vi "configure.vi"(8 "error in (no error)":errorcluster, 11 "user":string) -> (0 "error out":errorcluster, 2 "cancelled?":bool)   [LabVIEW 2010]
uses:
  components/Stage/GenericStage/GenericStage/GenericStage.lvclass
  components/ExperimentController/GenericExperimentController/GenericExperimentController/GenericExperimentController.lvclass
  components/ImagingMode/GenericImagingMode/GenericImagingMode/GenericImagingMode.lvclass
  components/Objective/GenericObjective/GenericObjective/GenericObjective.lvclass
  common/classes/ErrorController/ErrorController/class_data.vi
  common/classes/GenericComponent/GenericComponent/GenericComponent.lvclass
  common/classes/ErrorController/ErrorController/ErrorController.lvclass
panel:
  in  "Tab Control":T1(tab)
  in  "configure experiment controllers":bool
  in  "configure scan modes":bool
  in  "manageObjectivesButton":bool
  in  "configure objectives":bool
  in  "configure stage":bool
  in  "stage configuration":string(combo) caption="configuration"
  in  "stage path":path=path "C:/helioscan/plugins/scan_head/DL090202ScanHead/DL090202ScanHead/DL090202ScanHead.lvclass" caption="Component class path (.lvclass file)"
  in  "cancelButton":bool
  in  "save":bool
  # "HelioScan Main Configuration"
  # "ExperimentController components control the execution of individual scans. Here you can add ExperimentControllers, such that they can be selected from a drop-down menu in the main application. \n\nImportant: Note that some of the ExperimentControllers might require to be configured before you add them here."
  # "Each ImagingMode component controls a specific kind of image acquisition (e.g., video camera, intrinsic imaging, different laser-scanning-based ImagingModes, etc.). Here you can add ImagingModes, such that they can be selected from a drop-down menu in the main application. \n\nImportant: Note that you have to configure an ImagingMode before you can add it here."
  # "Objective components hold information about a specific microscope objective (e.g., magnification, manufacturer, etc.).\n\nImportant: Note that you have to configure an Objective component before you can add it here."
  # "The Stage component is responsible for controlling a motorised microscopy stage.\n\nNote: If you do not want to control a stage with HelioScan, just leave the input boxes below empty."
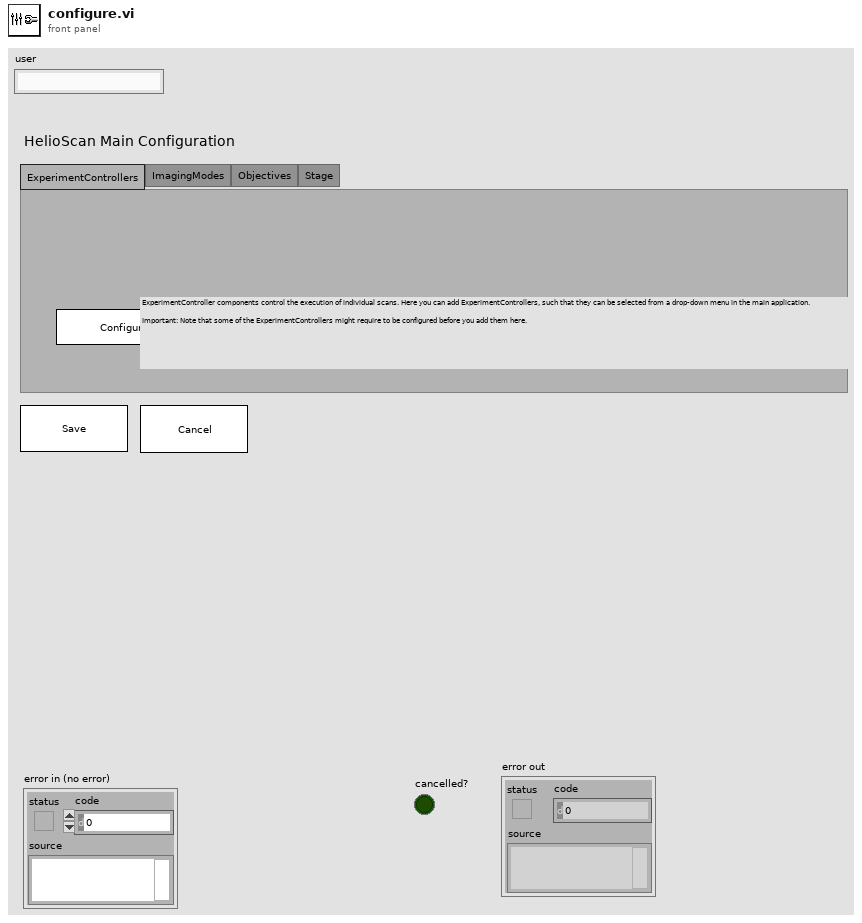
[diagram p1: front panel]
types:
  T1 = enum32{"ExperimentControllers", "ImagingModes", "Objectives", "Stage"}
  T2 = typedef "configuration_paths_cluster.ctl" = cluster{"base folder":path, "base folder for user":path, "component folder":path, "component file path":path, "main folder":path, "main file":path}
  T3 = typedef "top_level_config_cluster.ctl" = cluster{"experimentControllers":T4[], "default experimentController":string, "imagingModes":T4[], "default imagingMode":string, "stage":T4, "objectives":T4[], "default objective":string}
  T4 = typedef "plugin_specification.ctl" = cluster{"class path":string, "configuration":string, "label":string, "settings name":string}
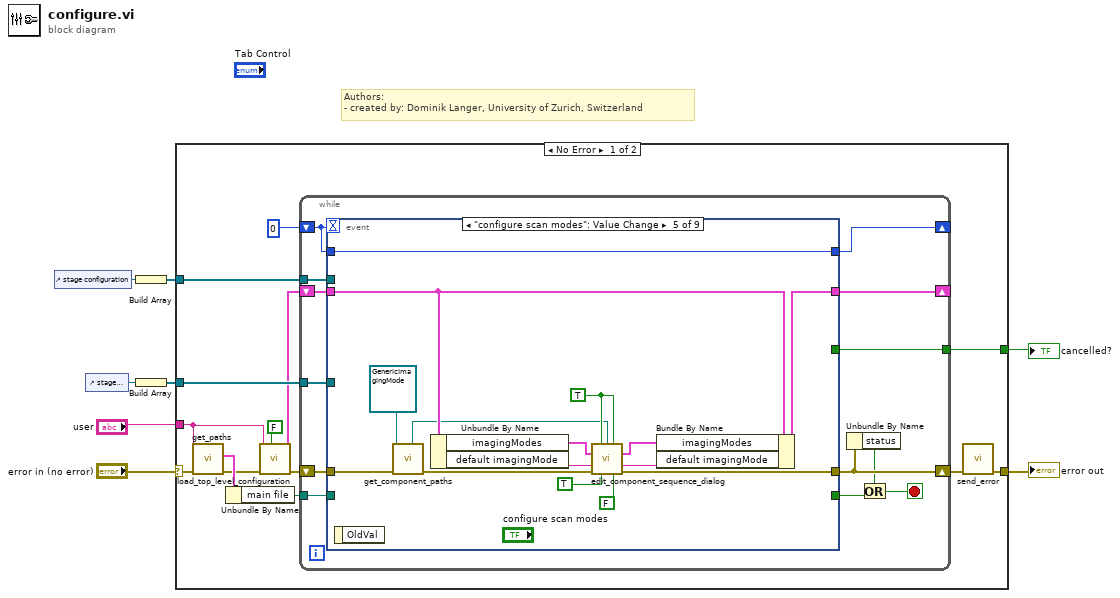
[diagram p0: block diagram]
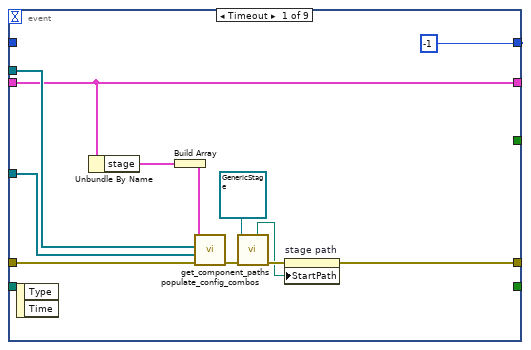
[diagram p2: hidden frame]
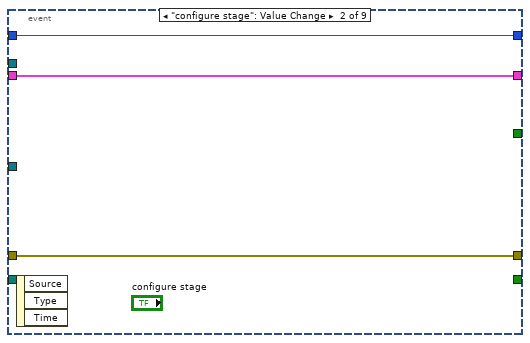
[diagram p3: hidden frame]
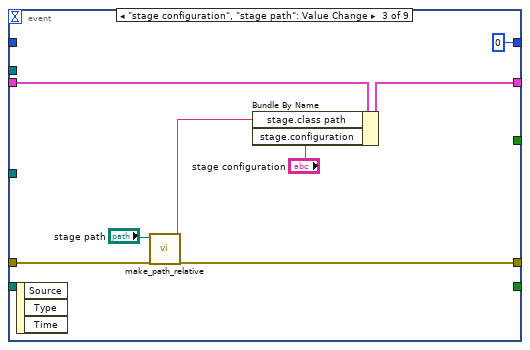
[diagram p4: hidden frame]
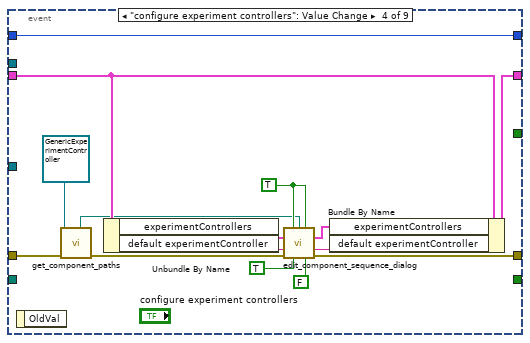
[diagram p5: hidden frame]
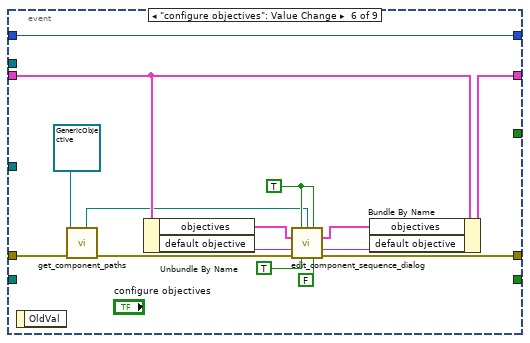
[diagram p6: hidden frame]
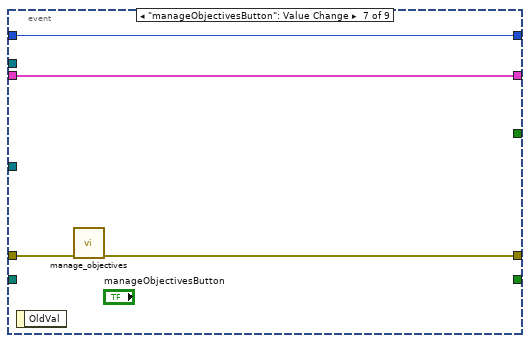
[diagram p7: hidden frame]
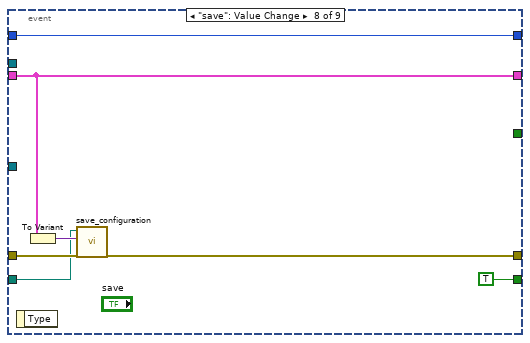
[diagram p8: hidden frame]
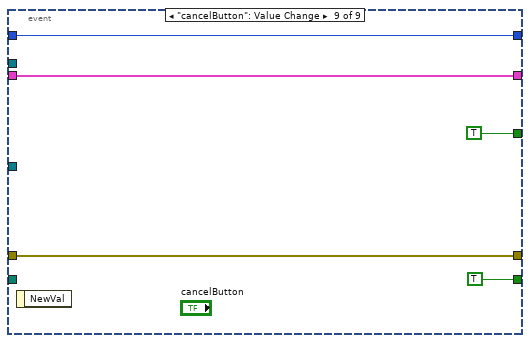
[diagram p9: hidden frame]
diagram:
  # "Authors: \n- created by: Dominik Langer, University of Zurich, Switzerland"
  n1 = control-ref of="stage configuration"() -> (w4:refnum<vi>)
  n2 = control-ref of="stage path"() -> (w3:refnum<vi>)
  n3 = Build Array(w4) -> (w6:refnum<vi>[])
  n4 = Build Array(w3) -> (w5:refnum<vi>[])
  n5 = case shown="No Error" "error in (no error)" {
    selector: "error in (no error)" -> [w19 w120]
    tunnel: [w9 w120] -> w7
    tunnel: w6 -> [w21 _]
    tunnel: w5 -> [w20 _]
    tunnel: "user" -> [w14 _]
    tunnel: [w11 _] -> w1
    frame No Error {
      n6 = call "get_paths.vi"("error in (no error)"=w19, "user"=w14) -> ("error out"=w16:errorcluster, "configuration paths"=w18:T2)  [unwired: 6 in, 2 out]
      n7 = Unbundle By Name(w18) -> ("main file"=w17:path)
      n8 = call "load_top_level_configuration.vi"("force load?"=FALSE, "error in (no error)"=w16, "user"=w14) -> ("error out"=w15:errorcluster, "configuration"=w12:T3)  [unwired: 7 in]
      n9 = while {
        shift-right: [w34] -> _
        shift-left: 0 -> [w35]
        shift-right: [w33] -> _
        shift-left: w12 -> [w31]
        tunnel: w21 -> [w30]
        tunnel: w20 -> [w29]
        tunnel: w17 -> [w24]
        tunnel: [w23] -> w11
        shift-right: [w28] -> w10
        shift-left: w15 -> [w32]
        stop <- w26 stop-if-true
        n10 = event shown="[4] \"configure scan modes\": Value Change" {
          selector: _ -> [_ _ _ _ _ _ _ _ _]
          dyn-events: _ -> [_ _ _ _ _ _ _ _ _]
          timeout: w35 -> [_ _ _ _ _ _ _ _ _]
          tunnel: [-1 w50 0 w73 w88 w103 w107 w114 w118] -> w34
          tunnel: w35 -> [_ w50 _ w73 w88 w103 w107 w114 w118]
          tunnel: [_ _ _ _ _ _ _ TRUE TRUE] -> w25
          tunnel: [w42 w49 w57 w68 w81 w96 w106 w113 w117] -> w33
          tunnel: [w36 w48 w53 w72 w83 w98 w104 w112 w116] -> w28
          tunnel: w32 -> [w45 w48 w54 w62 w75 w90 w105 w109 w116]
          tunnel: w31 -> [w42 w49 w58 w69 w82 w97 w106 w113 w117]
          tunnel: w30 -> [w44 _ _ _ _ _ _ _ _]
          tunnel: w29 -> [w43 _ _ _ _ _ _ _ _]
          tunnel: w24 -> [_ _ _ _ _ _ _ w108 _]
          tunnel: [_ _ _ _ _ _ _ _ TRUE] -> w23
          event Timeout {
            n11 = event-data() -> ()  [unwired: 3 out]
            n12 = Unbundle By Name(w42) -> ("stage"=w41:T4)
            n13 = Build Array(w41) -> (w46:T4[])
            n14 = call "populate_config_combos.vi"("error in (no error)"=w45, "plug-in path refs"=w43, "combo control refs"=w44, "configurations"=w46) -> ("error out"=w40:errorcluster)  [unwired: 7 out]
            n15 = call-dynamic "get_component_paths.vi"("error in (no error)"=w40, "GenericComponent in"=refnum<class "GenericStage.lvclass"> refnum ("GenericStage.lvclass")) -> ("error out"=w39:errorcluster, "component type directory"=w37:path)  [unwired: 4 in, 4 out]
            n16 = property on="stage path" class="Path"(error in=w39, "StartPath"=w37) -> (error out=w36:errorcluster)  [unwired: 1 in, 1 out]
          }
          event "configure stage": Value Change {
            n17 = event-data() -> ()  [unwired: 4 out]
          }
          event "stage configuration", "stage path": Value Change {
            n18 = event-data() -> ()  [unwired: 4 out]
            n19 = call "make_path_relative.vi"("error in (no error)"=w54, "absolute path"="stage path") -> ("error out"=w53:errorcluster, "relative path"=w51:string)  [unwired: 8 in]
            n20 = Bundle By Name(cluster=w58, "stage.class path"=w51, "stage.configuration"="stage configuration") -> (w57:T3)
          }
          event "configure experiment controllers": Value Change {
            w65 = TRUE ("show configuration?")
            n21 = event-data() -> ()  [unwired: 2 out]
            n22 = call-dynamic "get_component_paths.vi"("error in (no error)"=w62, "GenericComponent in"=refnum<class "GenericExperimentController.lvclass"> refnum ("GenericExperimentController.lvclass")) -> ("error out"=w61:errorcluster, "component type directory"=w59:path)  [unwired: 4 in, 4 out]
            n23 = Unbundle By Name(w69) -> ("experimentControllers"=w71:T4[], "default experimentController"=w70:string)
            n24 = call "edit_component_sequence_dialog.vi"("show configuration?"=w65, "default folder path"=w59, "show label?"=w65, "component specification list in"=w71, "default"=w70, "error in (no error)"=w61, "choose default?"=TRUE, "show settings?"=FALSE) -> ("component specification list out"=w66:T4[], "default"=w67:string, "error out"=w72:errorcluster)  [unwired: 5 in]
            n25 = Bundle By Name(cluster=w69, "experimentControllers"=w66, "default experimentController"=w67) -> (w68:T3)
          }
          event "configure scan modes": Value Change {
            w79 = TRUE ("show configuration?")
            n26 = event-data() -> ()  [unwired: 2 out]
            n27 = call-dynamic "get_component_paths.vi"("error in (no error)"=w75, "GenericComponent in"=refnum<class "GenericImagingMode.lvclass"> refnum ("GenericImagingMode.lvclass")) -> ("error out"=w74:errorcluster, "component type directory"=w77:path)  [unwired: 4 in, 4 out]
            n28 = Unbundle By Name(w82) -> ("imagingModes"=w87:T4[], "default imagingMode"=w86:string)
            n29 = call "edit_component_sequence_dialog.vi"("show configuration?"=w79, "default folder path"=w77, "show label?"=w79, "component specification list in"=w87, "default"=w86, "error in (no error)"=w74, "choose default?"=TRUE, "show settings?"=FALSE) -> ("component specification list out"=w84:T4[], "default"=w85:string, "error out"=w83:errorcluster)  [unwired: 5 in]
            n30 = Bundle By Name(cluster=w82, "imagingModes"=w84, "default imagingMode"=w85) -> (w81:T3)
          }
          event "configure objectives": Value Change {
            w95 = TRUE ("show configuration?")
            n31 = event-data() -> ()  [unwired: 2 out]
            n32 = call-dynamic "get_component_paths.vi"("error in (no error)"=w90, "GenericComponent in"=refnum<class "GenericObjective.lvclass"> refnum ("GenericObjective.lvclass")) -> ("error out"=w89:errorcluster, "component type directory"=w92:path)  [unwired: 4 in, 4 out]
            n33 = Unbundle By Name(w97) -> ("objectives"=w102:T4[], "default objective"=w101:string)
            n34 = call "edit_component_sequence_dialog.vi"("show configuration?"=w95, "default folder path"=w92, "show label?"=w95, "component specification list in"=w102, "default"=w101, "error in (no error)"=w89, "choose default?"=TRUE, "show settings?"=FALSE) -> ("component specification list out"=w99:T4[], "default"=w100:string, "error out"=w98:errorcluster)  [unwired: 5 in]
            n35 = Bundle By Name(cluster=w97, "objectives"=w99, "default objective"=w100) -> (w96:T3)
          }
          event "manageObjectivesButton": Value Change {
            n36 = event-data() -> ()  [unwired: 2 out]
            n37 = call "manage_objectives.vi"("error in (no error)"=w105) -> ("error out"=w104:errorcluster)  [unwired: 10 in]
          }
          event "save": Value Change {
            n38 = event-data() -> ()  [unwired: 2 out]
            n39 = To Variant(anything=w113) -> (Variant=w111:variant)
            n40 = call "save_configuration.vi"("error in (no error)"=w109, "config cluster variant in (data type)"=w111, "path"=w108) -> ("error out"=w112:errorcluster)  [unwired: 4 in, 4 out]
          }
          event "cancelButton": Value Change {
            n41 = event-data() -> ()  [unwired: 2 out]
          }
        }
        n42 = Unbundle By Name(w28) -> ("status"=w27:bool)
        n43 = Or(x=w27, y=w25) -> (x .or. y?=w26:bool)
      }
      n44 = call "send_error.vi"("error in (no error)"=w10) -> ("error out"=w9:errorcluster)  [unwired: 10 in]
    }
    frame Error {
    }
  }
  "error out" <- w7
  "cancelled?" <- w1
